vi "Begin.vi"(8 "error in":errorcluster) -> (0 "error out":errorcluster)   [LabVIEW 2018]
doc: "Called before other user functions, this VI can be used to open I/O refnums, load in file data, and do general program initialization. Notice that the <B>error out</B> terminal is simply used for data flow. Wiring it to other structures or subVIs ensures that this VI runs first."
uses:
  <vilib>/Rock Robotics/WPI/DriverStation/WPI_DriverStationRobotMode2.ctl
  <vilib>/Rock Robotics/WPI/Joystick/WPI_JoystickDeviceEnum.ctl
  <vilib>/Rock Robotics/SystemInterfaces/AI/FPGA_AIChannel.ctl
  <vilib>/Rock Robotics/SystemInterfaces/DIO/FPGA_DIOChannel.ctl
  Robot Global Data.vi
  <vilib>/Rock Robotics/Network Tables/NT Write String Array.vi
  <vilib>/Rock Robotics/WPI/Utilities/WPI_GetSetVariantRefNum.vi
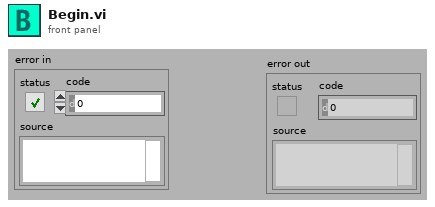
[diagram p1: front panel]
types:
  T1 = typedef "FPGA_DIOChannel.ctl" = enum8{"DIO 0", "DIO 1", "DIO 2", "DIO 3", "DIO 4", "DIO 5", "DIO 6", "DIO 7", "DIO 8", "DIO 9", "DIO MXP 0", "DIO MXP 1", "DIO MXP 2", "DIO MXP 3", "DIO MXP 4", "DIO MXP 5", "DIO MXP 6", "DIO MXP 7", "DIO MXP 8", "DIO MXP 9", "DIO MXP 10", "DIO MXP 11", "DIO MXP 12", "DIO MXP 13", "DIO MXP 14", "DIO MXP 15", "SPI Port CS1", "SPI Port CS2", "SPI Port CS3", "SPI Port MISO", "SPI Port MOSI", "Invalid"}
  T2 = typedef "WPI_JoystickDeviceEnum.ctl" = enum16{"USB 0", "USB 1", "USB 2", "USB 3", "USB 4", "USB 5"}
  T3 = typedef "FPGA_AIChannel.ctl" = enum8{"AI 0", "AI 1", "AI 2", "AI 3", "AI MXP 0", "AI MXP 1", "AI MXP 2", "AI MXP 3", "Invalid"}
  T4 = typedef "WPI_DriverStationRobotMode2.ctl" = enum16{"Autonomous Disabled", "Autonomous Enabled", "Teleop Disabled", "Teleop Enabled", "Disconnected", "Finish", "Test Disabled", "Test Enabled", "Emergency Stopped"}
  T5 = typedef "WPI_CompressorDevRef.ctl" = cluster{"DevStatus":errorcluster, "Pneumatics Control Module":u8}
  T6 = typedef "WPI_AnalogChannelDevRef.ctl" = cluster{"DevStatus":errorcluster, "Analog Channel":T3}
  T7 = typedef "WPI_JoystickDevRef.ctl" = cluster{"Device":T2}
  T8 = typedef "WPI_DigitalOutputDevRef.ctl" = cluster{"DIO Channel":T1, "DevStatus":errorcluster}
  T9 = typedef "WPI_DigitalInputDevRef.ctl" = cluster{"DevStatus":errorcluster, "DIO Channel":T1}
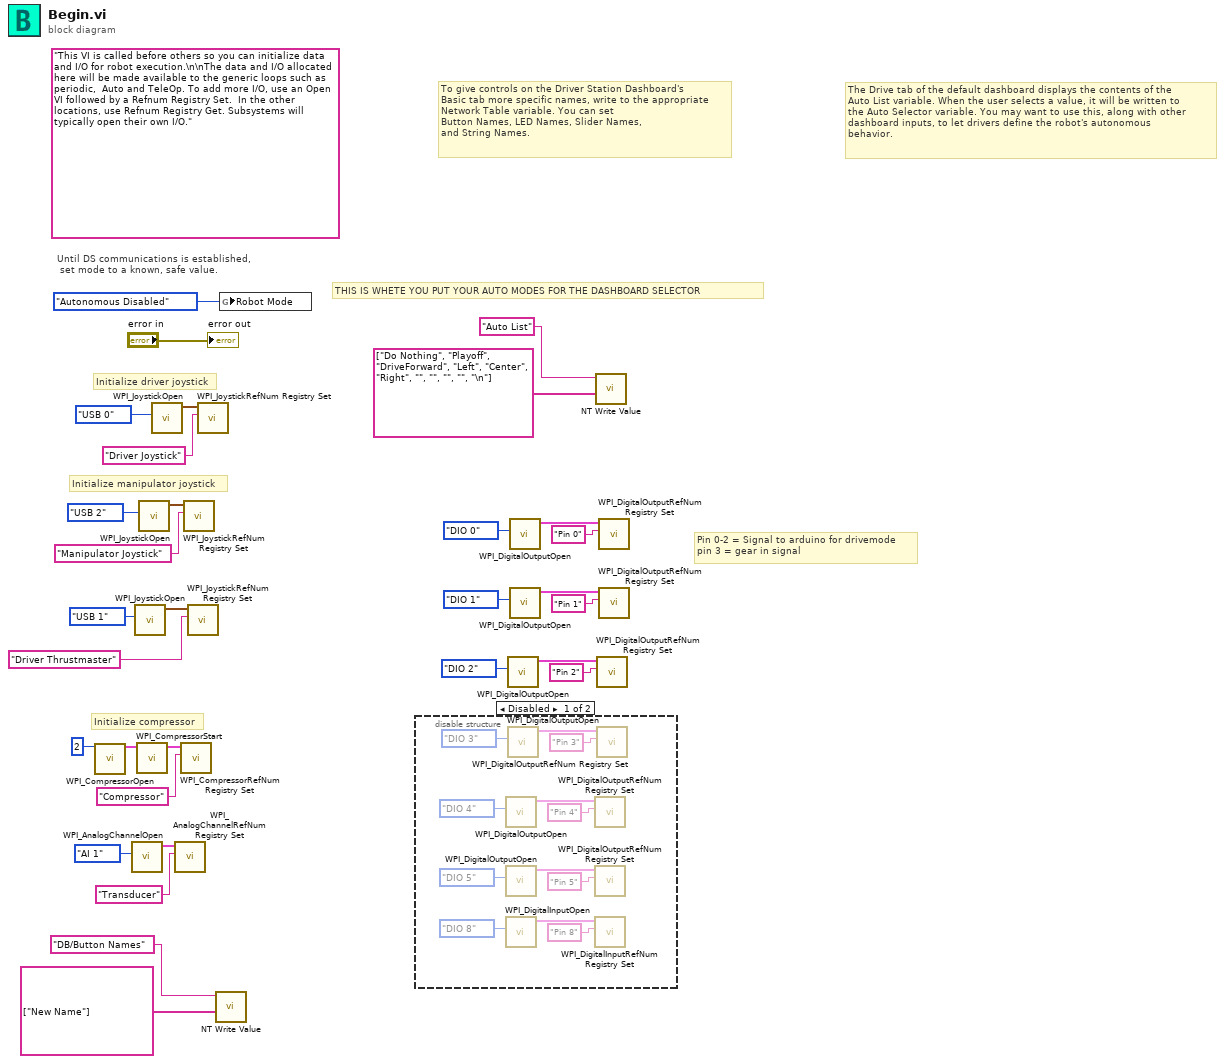
[diagram p0: block diagram]
diagram:
  (unwired) "This VI is called before others so you can initialize data and I/O for robot execution.\n\nThe data and I/O allocated here will be made available to the generic loops such as periodic,  Auto and TeleOp. To add more I/O, use an Open VI followed by a Refnum Registry Set.  In the other locations, use Refnum Registry Get. Subsystems will typically open their own I/O."
  # "Pin 0-2 = Signal to arduino for drivemode\npin 3 = gear in signal"
  # "Initialize compressor"
  # "Initialize manipulator joystick"
  # "THIS IS WHETE YOU PUT YOUR AUTO MODES FOR THE DASHBOARD SELECTOR"
  # "Initialize driver joystick"
  # "The Drive tab of the default dashboard displays the contents of the\nAuto List variable. When the user selects a value, it will be written to\nthe Auto Selector variable. You may want to use this, along with other\ndashboard inputs, to let drivers define the robot's autonomous\nbehavior."
  # "To give controls on the Driver Station Dashboard's\nBasic tab more specific names, write to the appropriate\nNetwork Table variable. You can set\nButton Names, LED Names, Slider Names,\nand String Names."
  # "Until DS communications is established,\n set mode to a known, safe value."
  n1 = call <vilib>:"WPI_CompressorOpen.vi"("Pneumatics Control Module (0)"=u8 2) -> ("CompressorDevRef"=w19:T5)  [unwired: 13 in, 1 out]
  n2 = call <vilib>:"WPI_AnalogChannelOpen.vi"("Analog Channel"=FPGA_AIChannel."AI 1") -> ("AIDeviceRef"=w13:T6)  [unwired: 9 in, 1 out]
  n3 = call <vilib>:"WPI_JoystickOpen.vi"("JoystickDevice"=WPI_JoystickDeviceEnum."USB 1") -> ("JoystickDevRef"=w11:T7)  [unwired: 10 in]
  n4 = call <vilib>:"WPI_CompressorStart.vi"("CompressorDevRef"=w19) -> ("CompressorDevRef"=w17:T5)  [unwired: 9 in, 1 out]
  n5 = call <vilib>:"WPI_JoystickOpen.vi"("JoystickDevice"=WPI_JoystickDeviceEnum."USB 2") -> ("JoystickDevRef"=w21:T7)  [unwired: 10 in]
  n6 = call <vilib>:"WPI_JoystickOpen.vi"("JoystickDevice"=WPI_JoystickDeviceEnum."USB 0") -> ("JoystickDevRef"=w24:T7)  [unwired: 10 in]
  n7 = call <vilib>:"WPI_AnalogChannelRefNum Registry Set.vi"("refnum name"="Transducer", "AIDeviceRef"=w13) -> ()  [unwired: 8 in, 2 out]
  n8 = call <vilib>:"WPI_CompressorRefNum Registry Set.vi"("refnum name"="Compressor", "CompressorDevRef"=w17) -> ()  [unwired: 8 in, 2 out]
  n9 = call <vilib>:"WPI_JoystickRefNum Registry Set.vi"("refnum name"="Manipulator Joystick", "JoystickDevRef"=w21) -> ()  [unwired: 8 in, 2 out]
  n10 = call <vilib>:"WPI_JoystickRefNum Registry Set.vi"("refnum name"="Driver Thrustmaster", "JoystickDevRef"=w11) -> ()  [unwired: 8 in, 2 out]
  n11 = call <vilib>:"WPI_JoystickRefNum Registry Set.vi"("refnum name"="Driver Joystick", "JoystickDevRef"=w24) -> ()  [unwired: 8 in, 2 out]
  n12 = call-poly <vilib>:"NT Write Value.vi"("String Array"=string[] ["New Name"], "Name"="DB/Button Names") -> ()  [unwired: 9 in, 1 out]
  n13 = global write "Robot Global Data.vi" "Robot Mode"(WPI_DriverStationRobotMode2."Autonomous Disabled" ("Robot Mode")) -> ()
  n14 = disable-structure shown="Disabled" {
    frame Disabled {
      n15 = call <vilib>:"WPI_DigitalOutputOpen.vi"("DIO Channel"=FPGA_DIOChannel."DIO 4") -> ("DigitalOutputDevRef"=w37:T8)  [unwired: 9 in, 1 out]
      n16 = call <vilib>:"WPI_DigitalOutputOpen.vi"("DIO Channel"=FPGA_DIOChannel."DIO 5") -> ("DigitalOutputDevRef"=w39:T8)  [unwired: 9 in, 1 out]
      n17 = call <vilib>:"WPI_DigitalInputOpen.vi"("DIO Channel"=FPGA_DIOChannel."DIO 8") -> ("DigitalInputDevRef"=w33:T9)  [unwired: 9 in, 1 out]
      n18 = call <vilib>:"WPI_DigitalOutputOpen.vi"("DIO Channel"=FPGA_DIOChannel."DIO 3") -> ("DigitalOutputDevRef"=w42:T8)  [unwired: 9 in, 1 out]
      n19 = call <vilib>:"WPI_DigitalOutputRefNum Registry Set.vi"("refnum name"="Pin 4", "DigitalOutputDevRef"=w37) -> ()  [unwired: 8 in, 2 out]
      n20 = call <vilib>:"WPI_DigitalOutputRefNum Registry Set.vi"("refnum name"="Pin 5", "DigitalOutputDevRef"=w39) -> ()  [unwired: 8 in, 2 out]
      n21 = call <vilib>:"WPI_DigitalInputRefNum Registry Set.vi"("refnum name"="Pin 8", "DigitalInputDevRef"=w33) -> ()  [unwired: 8 in, 2 out]
      n22 = call <vilib>:"WPI_DigitalOutputRefNum Registry Set.vi"("refnum name"="Pin 3", "DigitalOutputDevRef"=w42) -> ()  [unwired: 8 in, 2 out]
    }
    frame Enabled {
    }
  }
  n23 = call <vilib>:"WPI_DigitalOutputOpen.vi"("DIO Channel"=FPGA_DIOChannel."DIO 2") -> ("DigitalOutputDevRef"=w2:T8)  [unwired: 9 in, 1 out]
  n24 = call <vilib>:"WPI_DigitalOutputOpen.vi"("DIO Channel"=FPGA_DIOChannel."DIO 0") -> ("DigitalOutputDevRef"=w6:T8)  [unwired: 9 in, 1 out]
  n25 = call <vilib>:"WPI_DigitalOutputOpen.vi"("DIO Channel"=FPGA_DIOChannel."DIO 1") -> ("DigitalOutputDevRef"=w8:T8)  [unwired: 9 in, 1 out]
  n26 = call-poly <vilib>:"NT Write Value.vi"("String Array"=string[] ["Do Nothing", "Playoff", "DriveForward", "Left", "Center", "Right", "", "", "", "", "\n"], "Name"="Auto List") -> ()  [unwired: 9 in, 1 out]
  n27 = call <vilib>:"WPI_DigitalOutputRefNum Registry Set.vi"("refnum name"="Pin 2", "DigitalOutputDevRef"=w2) -> ()  [unwired: 8 in, 2 out]
  n28 = call <vilib>:"WPI_DigitalOutputRefNum Registry Set.vi"("refnum name"="Pin 0", "DigitalOutputDevRef"=w6) -> ()  [unwired: 8 in, 2 out]
  n29 = call <vilib>:"WPI_DigitalOutputRefNum Registry Set.vi"("refnum name"="Pin 1", "DigitalOutputDevRef"=w8) -> ()  [unwired: 8 in, 2 out]
  "error out" <- "error in"
